vi "Update Cycles.vi"(11 "cluster in":T1) -> (3 "cluster out":T1)   [LabVIEW 2026]
uses:
  Type Defs/Handler Data.ctl
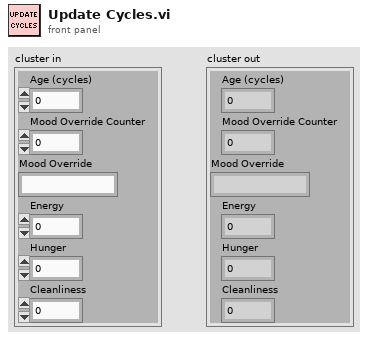
[diagram p1: front panel]
types:
  T1 = typedef "Handler Data.ctl" = cluster{"Age (cycles)":u32, "Mood Override Counter":u32, "Mood Override":string, "Energy":i16, "Hunger":i16, "Cleanliness":i16}
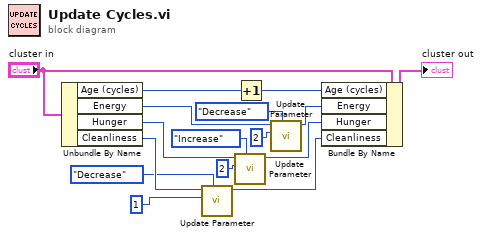
[diagram p0: block diagram]
diagram:
  n1 = Unbundle By Name("cluster in") -> ("Age (cycles)"=w8:u32, "Energy"=w11:i16, "Hunger"=w13:i16, "Cleanliness"=w15:i16)
  n2 = call "Update Parameter.vi"("Action"=enum16{"Increase", "Decrease"}."Decrease", "Modifier"=i16 1, "Parameter"=w15) -> ("New Value"=w16:i16)  [unwired: 8 in]
  n3 = call "Update Parameter.vi"("Action"=enum16{"Increase", "Decrease"}."Increase", "Modifier"=i16 2, "Parameter"=w13) -> ("New Value"=w14:i16)  [unwired: 8 in]
  n4 = Increment(x=w8) -> (x+1=w10:u32)
  n5 = call "Update Parameter.vi"("Action"=enum16{"Increase", "Decrease"}."Decrease", "Modifier"=i16 2, "Parameter"=w11) -> ("New Value"=w12:i16)  [unwired: 8 in]
  n6 = Bundle By Name(cluster="cluster in", "Age (cycles)"=w10, "Energy"=w12, "Hunger"=w14, "Cleanliness"=w16) -> (→"cluster out":T1)
